vi "Main.vi"(8 "error in":errorcluster, 11 "TCP Client Example in":refnum<class "TCP Client Example.lvclass">) -> (0 "error out":errorcluster, 3 "TCP Client Example out":refnum<class "TCP Client Example.lvclass">)   [LabVIEW 2017, in "TCP Client Example.lvclass"]
doc: "The <b>Queued Message Handler</b> of the Worker that owns this VI."
uses:
  TCP Client Example.lvclass
  C:/SC/Source Code/VIPM/LabVIEW 20xx/vi.lib/addons/_Workers/Library/Classes/Worker/Worker.lvclass
  Initialization Data.ctl
  TCP Client/TCP Client/Initialization Data.ctl
  TCP Client/TCP Client/Response Cases.ctl
  <vilib>/addons/_Workers/Library/Case Label.ctl
  TCP Client Example.lvclass/TCP Client Example.ctl
  TCP Client/TCP Client/rwr_Connect to Server.ctl
  TCP Client/TCP Client/rqp_Send String to Server.ctl
  <vilib>/addons/_Workers/Library/Classes/Message Queue/Message Queue.lvclass
  TCP Client/TCP Client/TCP Client.lvclass
  <vilib>/addons/_Workers/Library/Workers.lvlib
panel:
  out "Server name":string caption="Server Name"
  in  "Disconnect from Server":bool
  in  "Connect to Server":bool
  out "String Received from Server":string
  in  "String to Send to Server":string
  out "Connected?":bool
  in  "Server Port":u16=7654
  in  "Server IP Address":string="127.0.0.1"
  out "Client Name":string
  out "Title":string
  # "Server IP Address"
  # "Server Port"
  # "Connected? :"
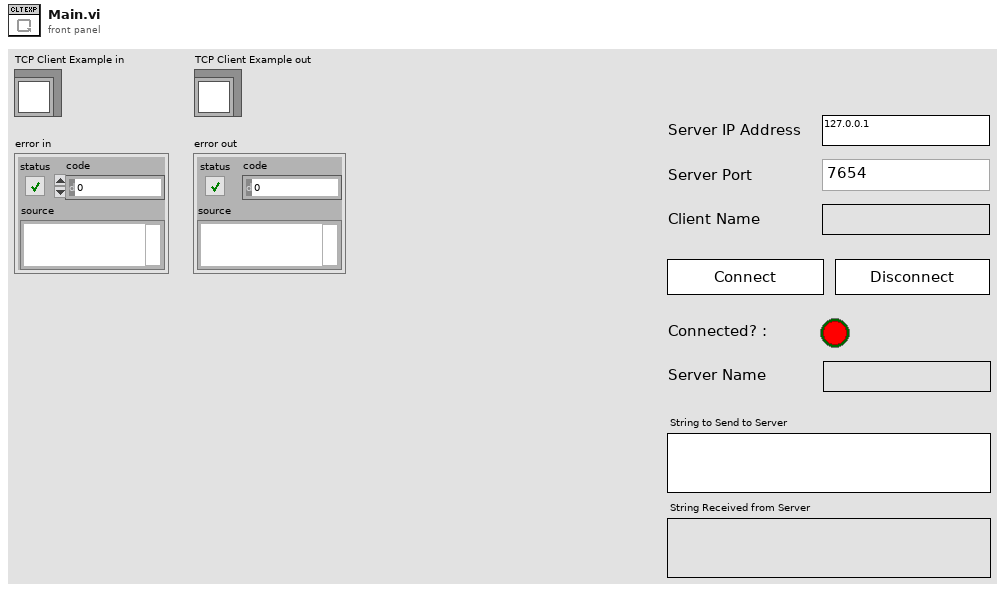
[diagram p1: front panel]
types:
  T1 = typedef "TCP Client Example.lvclass/Initialization Data.ctl" = cluster{"Client Name":string}
  T2 = typedef "_TCP Client.lvlib/TCP Client.lvclass/Initialization Data.ctl" = cluster{"Response Cases":T3}
  T3 = typedef "_TCP Client.lvlib/TCP Client.lvclass/Response Cases.ctl" = cluster{"Connection Notify":T4, "Incoming Data":T4}
  T4 = typedef "Workers.lvlib/Case Label.ctl" = string
  T5 = typedef "_TCP Client.lvlib/TCP Client.lvclass/rwr_Connect to Server.ctl" = cluster{"Client Name":string, "Server IP Address":string, "Server Port":u16}
  T6 = typedef "_TCP Client.lvlib/TCP Client.lvclass/rqp_Send String to Server.ctl" = cluster{"String to Send":string}
  T7 = typedef "_TCP Client.lvlib/TCP Client.lvclass/rsp_Connection Notify.ctl" = cluster{"Server Name":string, "IP Address":string, "Connected?":bool}
  T8 = typedef "_TCP Client.lvlib/TCP Client.lvclass/rsp_Incoming Data.ctl" = cluster{"Data":string}
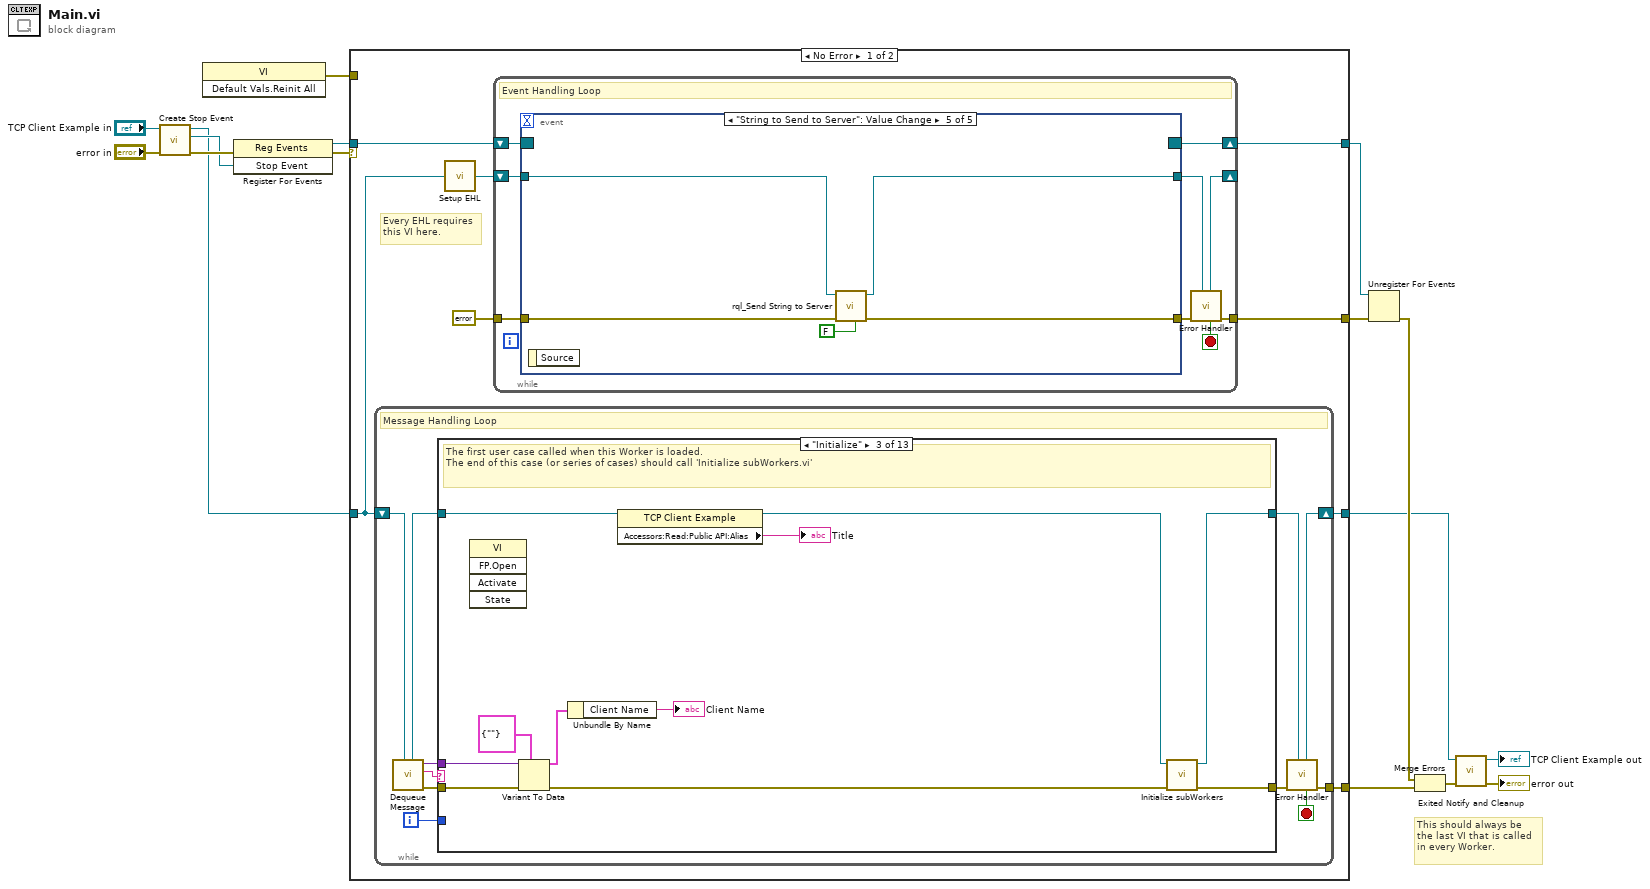
[diagram p0: block diagram]
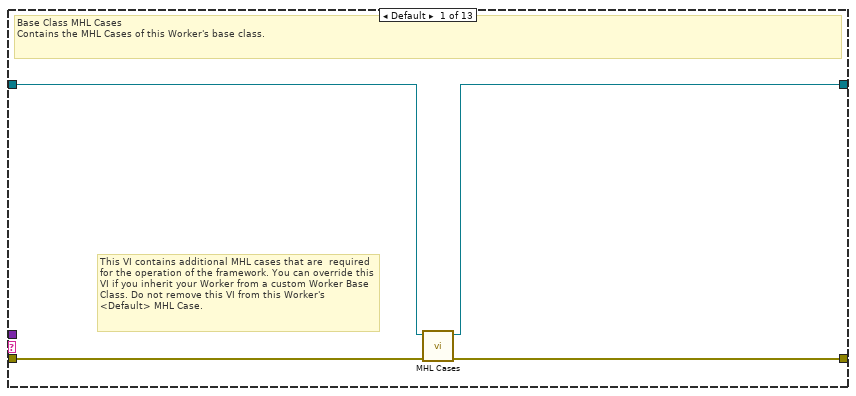
[diagram p2: hidden frame]
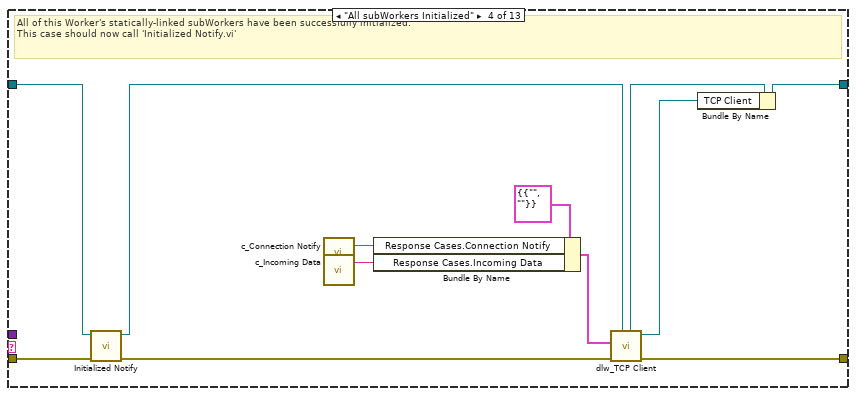
[diagram p4: hidden frame]
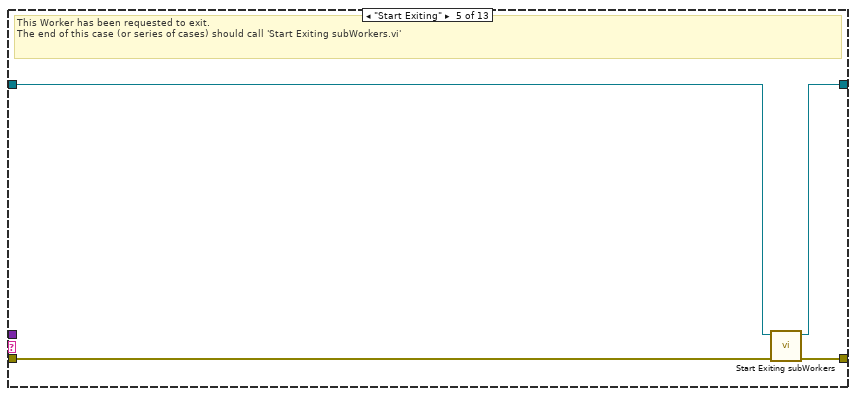
[diagram p5: hidden frame]
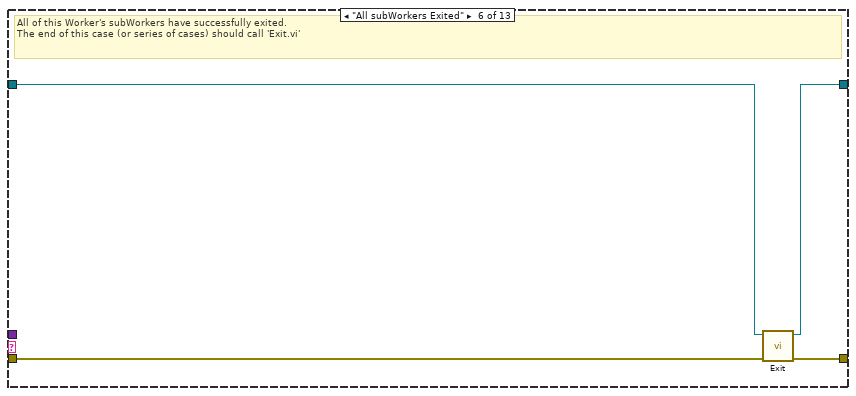
[diagram p6: hidden frame]
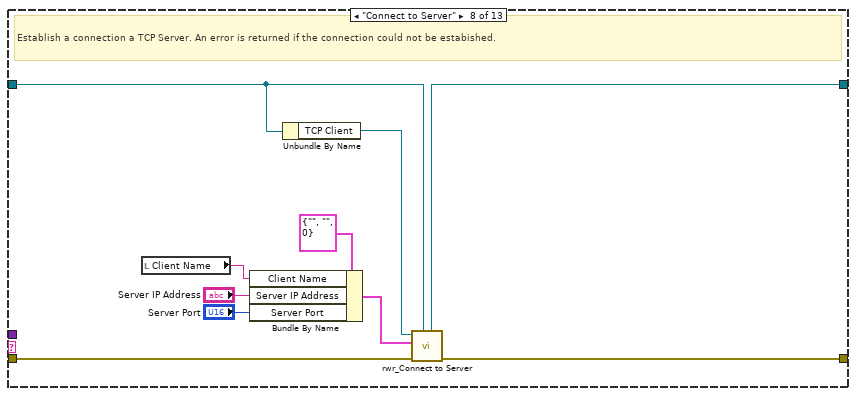
[diagram p8: hidden frame]
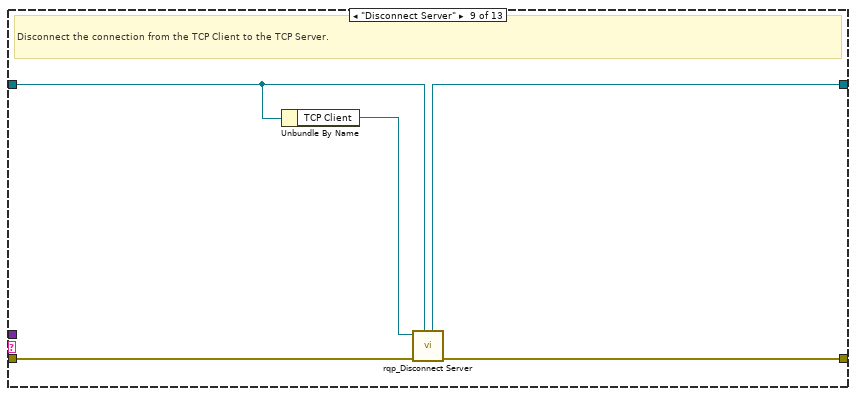
[diagram p9: hidden frame]
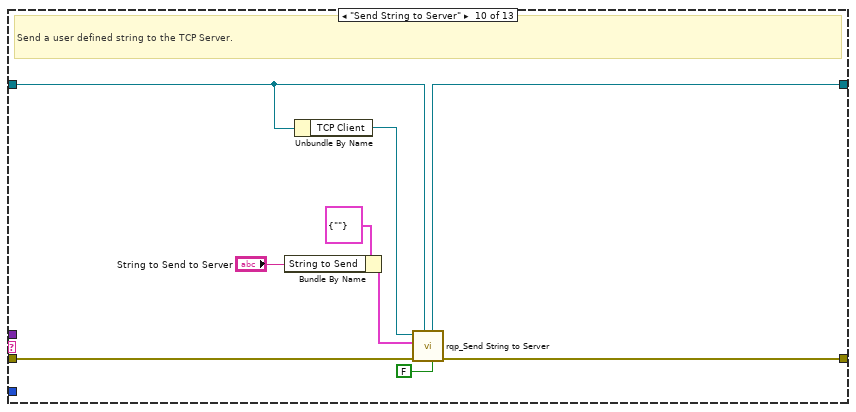
[diagram p10: hidden frame]
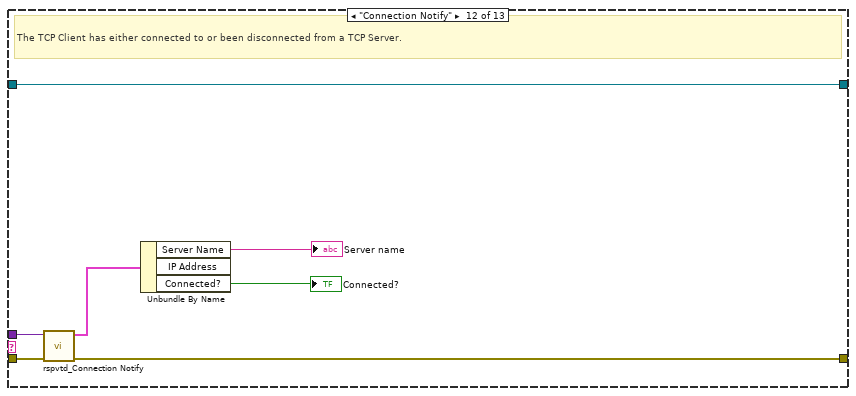
[diagram p12: hidden frame]
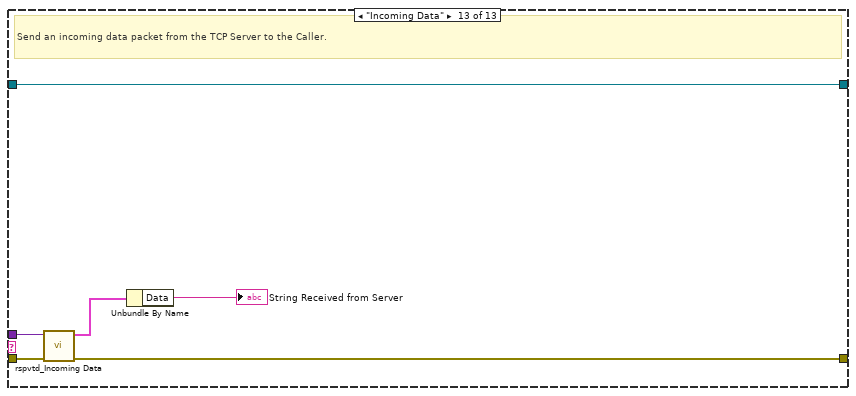
[diagram p13: hidden frame]
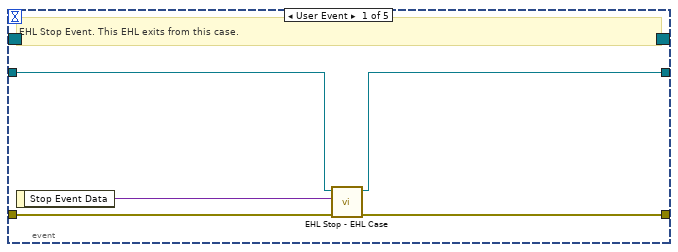
[diagram p14: hidden frame]
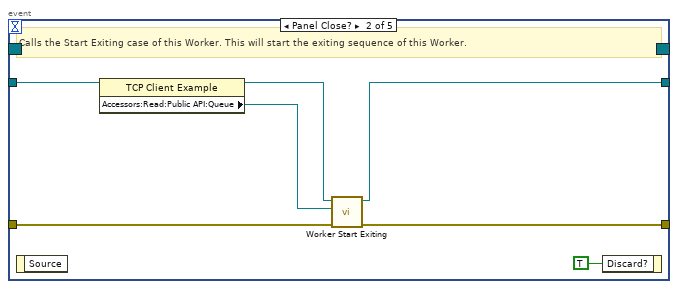
[diagram p15: hidden frame]
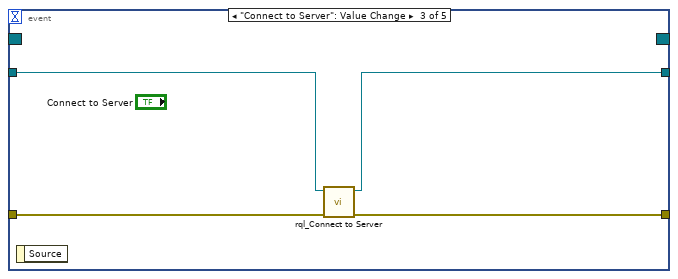
[diagram p16: hidden frame]
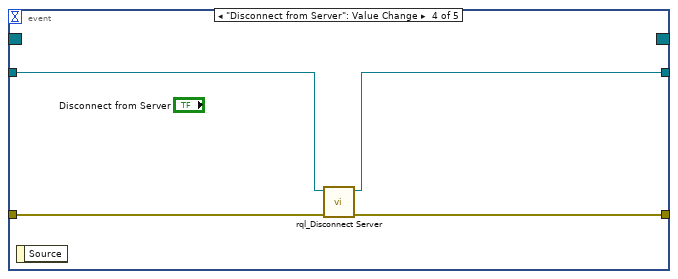
[diagram p17: hidden frame]
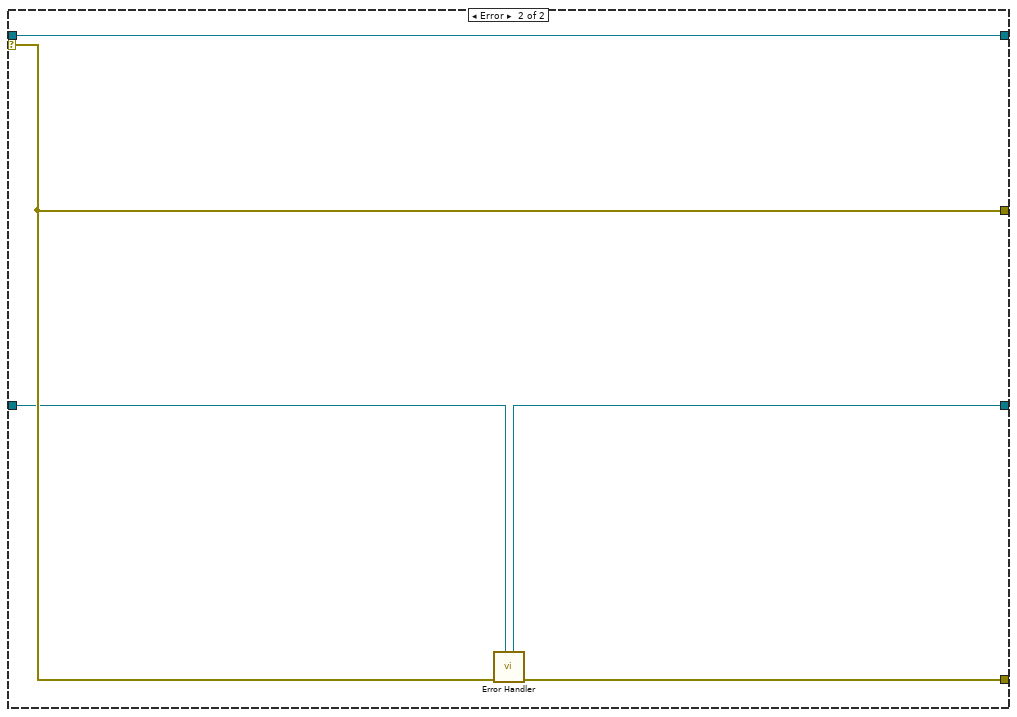
[diagram p18: hidden frame]
diagram:
  # "This should always be the last VI that is called in every Worker."
  n1 = call-dynamic "Create Stop Event.vi"("error in"="error in", "Worker"="TCP Client Example in") -> ("error out"=w11:errorcluster, "Stop Event"=w8:refnum<user-event>, "Worker out"=w5:refnum<class "TCP Client Example.lvclass">)  [unwired: 7 in]
  n2 = invoke class="VI" method="Default Vals.Reinit All"() -> (error out=w3:errorcluster)  [unwired: 3 in, 2 out]
  n3 = register-events(error in=w11, w8) -> (reference out=w10:refnum<event-registration>, error out=w4:errorcluster)  [unwired: 1 in]
  n4 = case shown="No Error" w4 {
    tunnel: w5 -> [w19 w149]
    tunnel: [w17 w150] -> w9
    tunnel: w10 -> [w24 w151]
    tunnel: [w21 w152] -> w15
    tunnel: [w23 w151] -> w14
    tunnel: [w18 w148] -> w12
    selector: w4 -> [_ w152]
    tunnel: w3 -> [_ _]
    frame No Error {
      # "Every EHL requires\nthis VI here."
      n5 = while {
        shift-right: [w33] -> w18
        shift-left: w19 -> [w35]
        tunnel: [w34] -> w17
        i -> [w26]
        stop <- w27 stop-if-true
        # "Message Handling Loop"
        n6 = call-dynamic "Dequeue Message.vi"("Worker"=w35) -> ("error out"=w32:errorcluster, "Case out"=w28:string, "Data out"=w25:variant, "Worker out"=w30:refnum<class "TCP Client Example.lvclass">)  [unwired: 6 in, 1 out]
        n7 = case "Worker MHL Case Structure (DO NOT CHANGE LABEL NAME)" shown="\"Initialize\"" w28 {
          tunnel: w32 -> [w39 w40 w50 w63 w65 w72 w74 w84 w89 w98 w100 w107 w113]
          tunnel: [w38 w40 w52 w60 w68 w71 w74 w83 w88 w97 w100 w105 w111] -> w31
          tunnel: w30 -> [w37 w41 w45 w64 w66 w70 w73 w76 w86 w95 w99 w106 w112]
          tunnel: [w36 w41 w51 w56 w67 w69 w73 w82 w87 w96 w99 w106 w112] -> w29
          tunnel: w26 -> [_ _ _ _ _ _ _ _ _ _ _ _ _]
          tunnel: w25 -> [_ _ w48 _ _ _ _ _ _ _ _ w104 w110]
          frame Default {
            # "This VI contains additional MHL cases that are  required for the operation of the framework. You can override this VI if you inherit your Worker from a custom Worker Base Class. Do not remove this VI from this Worker's <Default> MHL Case."
            # "Base Class MHL Cases\nContains the MHL Cases of this Worker's base class."
            n8 = call-dynamic "MHL Cases.vi"("error in"=w39, "Worker in"=w37) -> ("error out"=w38:errorcluster, "Worker out"=w36:refnum<class "TCP Client Example.lvclass">)  [unwired: 8 in]
          }
          frame "------------ FRAMEWORK CASES -----------" {
            # "Start of Workers Framework Cases"
          }
          frame "Initialize" {
            # "The first user case called when this Worker is loaded.\nThe end of this case (or series of cases) should call 'Initialize subWorkers.vi'"
            n9 = invoke class="VI" method="FP.Open"() -> ()  [unwired: 5 in, 5 out]
            n10 = Variant To Data(error in=w50, type=T1 {"Client Name"=""} ("Initialization Data"), Variant=w48) -> (data=w46:T1, error out=w49:errorcluster)
            n11 = Unbundle By Name(w46) -> ("Client Name"=→"Client Name":string)
            n12 = property class="TCP Client Example"(reference=w45) -> (reference out=w43:refnum<class "TCP Client Example.lvclass">, "Accessors:Read:Public API:Alias"=→"Title":string)  [unwired: 1 in, 1 out]
            n13 = call-dynamic "Initialize subWorkers.vi"("error in"=w49, "Worker"=w43) -> ("error out"=w52:errorcluster, "dup Worker out"=w51:refnum<class "TCP Client Example.lvclass">)  [unwired: 8 in]
          }
          frame "All subWorkers Initialized" {
            # "All of this Worker's statically-linked subWorkers have been successfully initialized.\nThis case should now call 'Initialized Notify.vi'"
            n14 = call-dynamic "Initialized Notify.vi"("error in"=w63, "Worker"=w64) -> ("error out"=w62:errorcluster, "dup Worker out"=w61:refnum<class "TCP Client Example.lvclass">)  [unwired: 8 in]
            n15 = call "c_Connection Notify.vi"() -> ("Case Label"=w54:T4)  [unwired: 1 in]
            n16 = call "c_Incoming Data.vi"() -> ("Case Label"=w53:T4)  [unwired: 1 in]
            n17 = Bundle By Name(cluster=T2 {"Response Cases"={"Connection Notify"="", "Incoming Data"=""}} ("Initialization Data"), "Response Cases.Connection Notify"=w54, "Response Cases.Incoming Data"=w53) -> (w57:T2)
            n18 = call "dlw_TCP Client.vi"("Caller in"=w61, "error in"=w62, "Initialization Data"=w57) -> ("error out"=w60:errorcluster, "TCP Client out"=w55:refnum<class "TCP Client.lvclass">, "dup Caller out"=w59:refnum<class "TCP Client Example.lvclass">)  [unwired: 6 in]
            n19 = Bundle By Name(cluster=w59, "TCP Client"=w55) -> (w56:refnum<class "TCP Client Example.lvclass">)
          }
          frame "Start Exiting" {
            # "This Worker has been requested to exit. \nThe end of this case (or series of cases) should call 'Start Exiting subWorkers.vi'"
            n20 = call-dynamic "Start Exiting subWorkers.vi"("error_in"=w65, "Worker"=w66) -> ("error out"=w68:errorcluster, "dup Worker out"=w67:refnum<class "TCP Client Example.lvclass">)  [unwired: 8 in]
          }
          frame "All subWorkers Exited" {
            # "All of this Worker's subWorkers have successfully exited. \nThe end of this case (or series of cases) should call 'Exit.vi'"
            n21 = call-dynamic "Exit.vi"("error_in"=w72, "Worker"=w70) -> ("error out"=w71:errorcluster, "dup Worker out"=w69:refnum<class "TCP Client Example.lvclass">)  [unwired: 8 in]
          }
          frame "------------- LOCAL API CASES -------------" {
            # "Start of Workers Local API Cases"
          }
          frame "Connect to Server" {
            # "Establish a connection a TCP Server. An error is returned if the connection could not be estabished."
            n22 = local read "Client Name"() -> (w78:string)
            n23 = Bundle By Name(cluster=T5 {"Client Name"="", "Server IP Address"="", "Server Port"=0} ("Connect to Server Data"), "Client Name"=w78, "Server IP Address"="Server IP Address", "Server Port"="Server Port") -> (w77:T5)
            n24 = Unbundle By Name(w76) -> ("TCP Client"=w75:refnum<class "TCP Client.lvclass">)
            n25 = call "rwr_Connect to Server.vi"("Caller in"=w76, "error in"=w84, "Data in"=w77, "TCP Client in"=w75) -> ("error out"=w83:errorcluster, "dup Caller out"=w82:refnum<class "TCP Client Example.lvclass">)  [unwired: 4 in, 2 out]
          }
          frame "Disconnect Server" {
            # "Disconnect the connection from the TCP Client to the TCP Server."
            n26 = Unbundle By Name(w86) -> ("TCP Client"=w85:refnum<class "TCP Client.lvclass">)
            n27 = call "rqp_Disconnect Server.vi"("Caller in"=w86, "error in"=w89, "TCP Client in"=w85) -> ("error out"=w88:errorcluster, "dup Caller out"=w87:refnum<class "TCP Client Example.lvclass">)  [unwired: 6 in, 1 out]
          }
          frame "Send String to Server" {
            # "Send a user defined string to the TCP Server."
            n28 = Bundle By Name(cluster=T6 {"String to Send"=""} ("Data in"), "String to Send"="String to Send to Server") -> (w92:T6)
            n29 = Unbundle By Name(w95) -> ("TCP Client"=w94:refnum<class "TCP Client.lvclass">)
            n30 = call "rqp_Send String to Server.vi"("Show in Debugger?"=FALSE, "Caller in"=w95, "error in"=w98, "Data in"=w92, "TCP Client in"=w94) -> ("error out"=w97:errorcluster, "dup Caller out"=w96:refnum<class "TCP Client Example.lvclass">)  [unwired: 4 in, 1 out]
          }
          frame "------------- RESPONSE CASES --------------" {
            # "Start of Workers Response Cases"
          }
          frame "Connection Notify" {
            # "The TCP Client has either connected to or been disconnected from a TCP Server."
            n31 = call "rspvtd_Connection Notify.vi"("error in"=w107, "Data in"=w104) -> ("error out"=w105:errorcluster, "Data out"=w101:T7)  [unwired: 8 in]
            n32 = Unbundle By Name(w101) -> ("Server Name"=→"Server name":string, "Connected?"=→"Connected?":bool)  [unwired: 1 out]
          }
          frame "Incoming Data" {
            # "Send an incoming data packet from the TCP Server to the Caller."
            n33 = call "rspvtd_Incoming Data.vi"("error in"=w113, "Data in"=w110) -> ("error out"=w111:errorcluster, "Data out"=w109:T8)  [unwired: 8 in]
            n34 = Unbundle By Name(w109) -> ("Data"=→"String Received from Server":string)
          }
        }
        n35 = call-dynamic "Error Handler.vi"("Worker"=w29, "error_in"=w31) -> ("error out"=w34:errorcluster, "Stop Loop"=w27:bool, "Worker out"=w33:refnum<class "TCP Client Example.lvclass">)  [unwired: 7 in]
      }
      n36 = call-dynamic "Setup EHL.vi"("Worker"=w19) -> ("Worker out"=w20:refnum<class "TCP Client Example.lvclass">)  [unwired: 14 in]
      n37 = while "Event Handling Loop" {
        shift-right: [w122] -> w23
        shift-left: w24 -> [w121]
        tunnel: [w117] -> w21
        tunnel: errorcluster {"status"=FALSE, "code"=0, "source"=""} ("error constant") -> [w119]
        shift-right: [w115] -> _
        shift-left: w20 -> [w120]
        stop <- w114 stop-if-true
        # "Event Handling Loop"
        n38 = event shown="[4] \"String to Send to Server\": Value Change" {
          selector: w121 -> [_ _ _ _ _]
          dyn-events: [_ _ _ _ _] -> w122
          timeout: _ -> [_ _ _ _ _]
          tunnel: [w126 w133 w137 w141 w146] -> w118
          tunnel: w119 -> [w127 w132 w138 w142 w147]
          tunnel: w120 -> [w125 w131 w136 w140 w145]
          tunnel: [w124 w130 w135 w139 w144] -> w116
          event User Event {
            # "EHL Stop Event. This EHL exits from this case."
            n39 = event-data() -> ("Stop Event Data"=w123:variant)  [unwired: 1 in]
            n40 = call-dynamic "EHL Stop - EHL Case.vi"("error in"=w127, "Stop Event Data"=w123, "Worker"=w125) -> ("error out"=w126:errorcluster, "Worker out"=w124:refnum<class "TCP Client Example.lvclass">)  [unwired: 7 in]
          }
          event Panel Close? {
            # "Calls the Start Exiting case of this Worker. This will start the exiting sequence of this Worker."
            n41 = event-data() -> ()  [unwired: 1 in, 1 out]
            n42 = property class="TCP Client Example"(reference=w131) -> (reference out=w129:refnum<class "TCP Client Example.lvclass">, "Accessors:Read:Public API:Queue"=w128:refnum<class "Message Queue.lvclass">)  [unwired: 1 in, 1 out]
            n43 = call-dynamic "Worker Start Exiting.vi"("error_in"=w132, "Message Queue"=w128, "Worker"=w129) -> ("error out"=w133:errorcluster, "dup Worker out"=w130:refnum<class "TCP Client Example.lvclass">)  [unwired: 7 in]
            n44 = event-data ("Event Filter Node")("Discard?"=TRUE) -> ()  [unwired: 1 in, 1 out]
          }
          event "Connect to Server": Value Change {
            n45 = event-data() -> ()  [unwired: 1 in, 1 out]
            n46 = call "rql_Connect to Server.vi"("error in"=w138, "TCP Client Example in"=w136) -> ("error out"=w137:errorcluster, "dup TCP Client Example out"=w135:refnum<class "TCP Client Example.lvclass">)  [unwired: 8 in]
          }
          event "Disconnect from Server": Value Change {
            n47 = event-data() -> ()  [unwired: 1 in, 1 out]
            n48 = call "rql_Disconnect Server.vi"("error in"=w142, "TCP Client Example in"=w140) -> ("error out"=w141:errorcluster, "dup TCP Client Example out"=w139:refnum<class "TCP Client Example.lvclass">)  [unwired: 8 in]
          }
          event "String to Send to Server": Value Change {
            n49 = event-data() -> ()  [unwired: 1 in, 1 out]
            n50 = call "rql_Send String to Server.vi"("Show in Debugger?"=FALSE, "error in"=w147, "TCP Client Example in"=w145) -> ("error out"=w146:errorcluster, "dup TCP Client Example out"=w144:refnum<class "TCP Client Example.lvclass">)  [unwired: 7 in]
          }
        }
        n51 = call-dynamic "Error Handler.vi"("Worker"=w116, "error_in"=w118) -> ("error out"=w117:errorcluster, "Stop Loop"=w114:bool, "Worker out"=w115:refnum<class "TCP Client Example.lvclass">)  [unwired: 7 in]
      }
    }
    frame Error {
      n52 = call-dynamic "Error Handler.vi"("Worker"=w149, "error_in"=w152) -> ("error out"=w150:errorcluster, "Worker out"=w148:refnum<class "TCP Client Example.lvclass">)  [unwired: 7 in, 1 out]
    }
  }
  n53 = Unregister For Events(event registration refnum=w14, error in=w15) -> (error out=w16:errorcluster)
  n54 = Merge Errors(w16, w9) -> (w13:errorcluster)
  n55 = call-dynamic "Exited Notify and Cleanup.vi"("error_in"=w13, "Worker"=w12) -> ("error out"=→"error out":errorcluster, "dup Worker out"=→"TCP Client Example out":refnum<class "TCP Client Example.lvclass">)  [unwired: 8 in]
